vi "select edge test.vi"() -> ()   [LabVIEW 2018]
uses:
  Classes/Controller/Camera/Camera.lvclass
  <vilib>/vision/NI_Vision_Development_Module.lvlib
  <vilib>/vision/Image Controls.llb/IMAQ Image.ctl
  Classes/Controller/Camera/Material.ctl
  Classes/Controller/Camera/Camera settings.ctl
  Classes/Controller/Camera/Image processing.ctl
  Classes/Controller/Camera/Machine Vision.ctl
panel:
  out "array":sgl[](array[numeric])
  in  "Record point":bool
  out "Image Dst Out":T1
  out "Real World Coordinates":cluster{"X":sgl, "Y":sgl} {"Y" format="%.2f"; "X" format="%.2f"}
  out "Array of Real World Coordinates":cluster{"X":sgl, "Y":sgl}[](array[cluster]) {"Y" format="%.2f"; "X" format="%.2f"}
  out "Array":dbl[][](array[numeric])
  in  "Record line":bool
  in  "Stop":bool
  out "Image":T1(plugin-control)
  out "Camera":dbl[](array[numeric])
  in  "Machine Vision":T2
  in  "Image processing":T3={"Brightness"=128.0, "Contrast"=45.0, "Gamma"=1.0471123} {"Brightness" scale=0.0..400.0; "Contrast" scale=0.0..90.0; "Gamma" scale=0.005..5.0}
  in  "Camera settings":T4={"Gamma"=1.6, "Gain"=0, "Sharpness"=0, "Contrast"=0.0, "Exposure"=0.0078125} {"Exposure" min=0.000244140625 max=0.5 scale=0.0002..0.5; "Contrast" min=0.0 max=1.0 scale=0.0..1.0; "Sharpness" min=0 max=2 step=1 scale=0.0..2.0; "Gain" min=0 max=100 step=1 scale=0.0..100.0; "Gamma" min=0.01 max=10.0 scale=0.01..10.0}
  in  "Override presets":bool
  in  "Material":T5
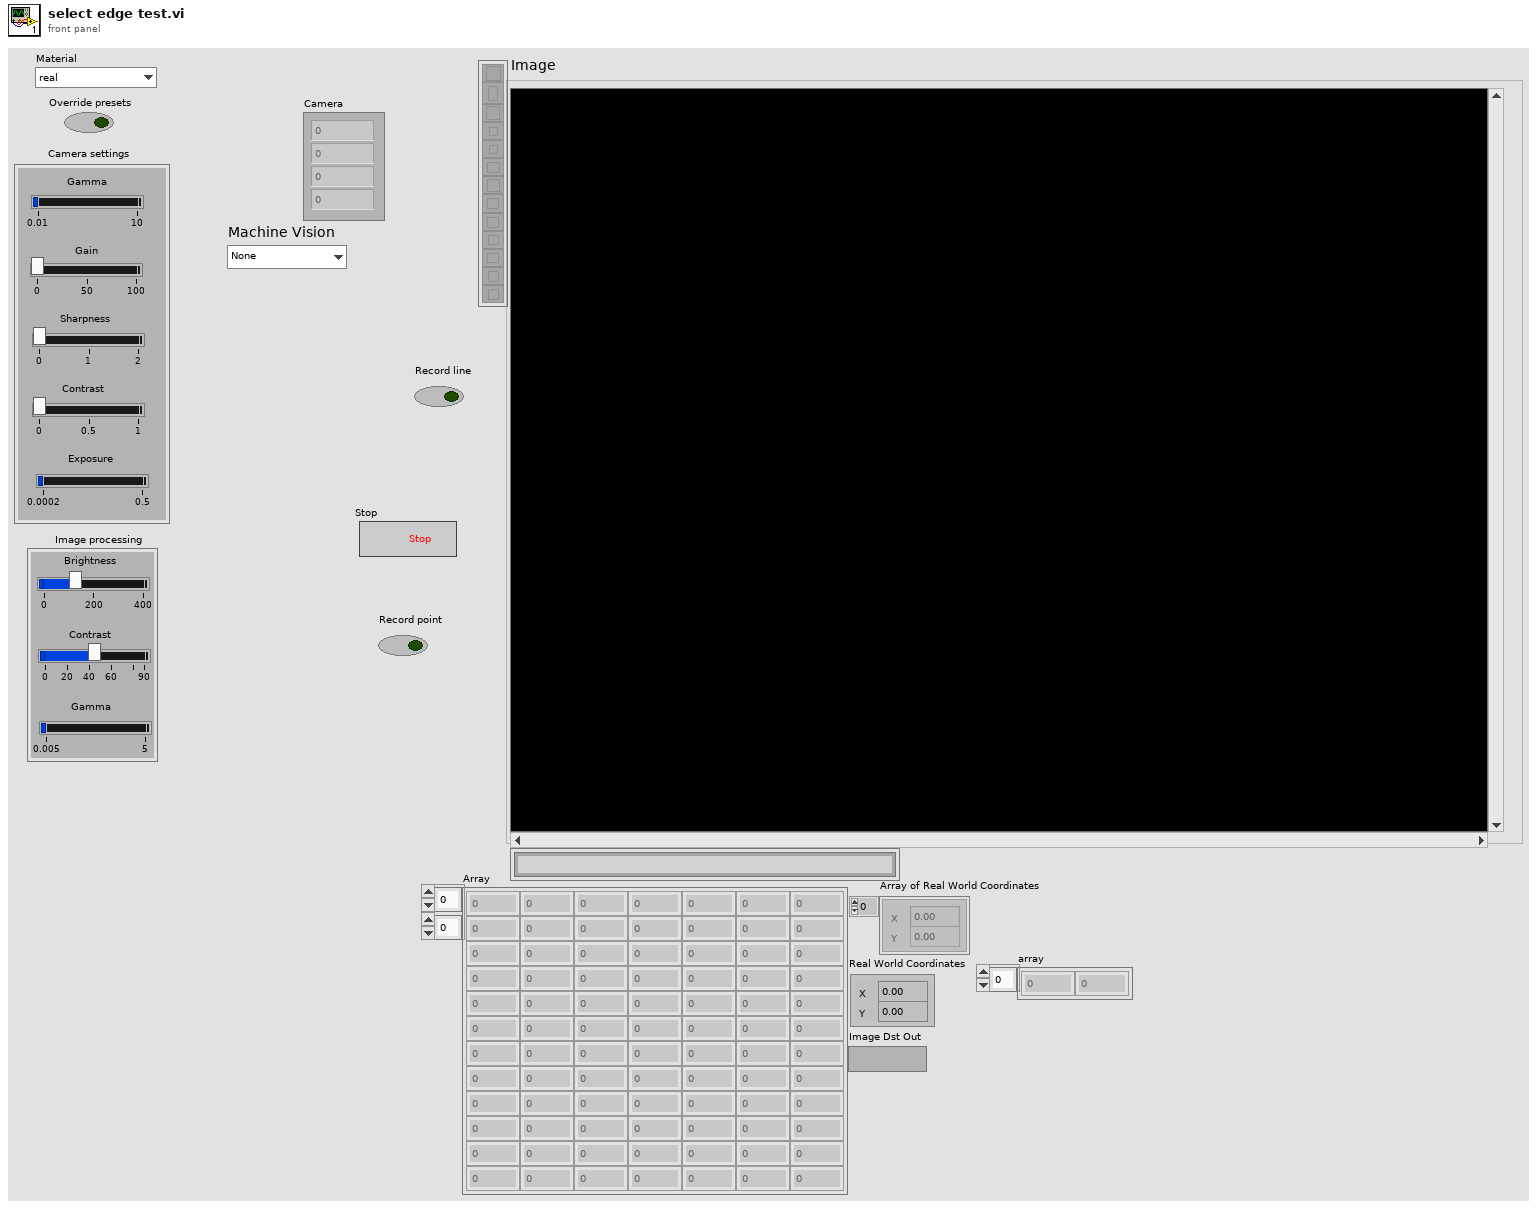
[diagram p1: front panel]
types:
  T1 = typedef "IMAQ Image.ctl" = refnum<image>
  T2 = typedef "Camera.lvclass/Machine Vision.ctl" = enum16{"None", "Tray Fiducials", "HPK Silicon", "100um dot", "Hexaboard", "Corner (TL, BR)", "Corner (BL, TR)", "BP gold pad 1", "BP gold pad 2", "BP gold pad 3", "dummy sensor CH2", "dummy sensor CH7", "dummy sensor CH191", "dummy sensor CH197", "sensor box", "sensor circle", "PCB PETG CH2", "PCB PETG CH7", "PCB PETG CH191", "PCB PETG CH197"}
  T3 = typedef "Camera.lvclass/Image processing.ctl" = cluster{"Brightness":sgl, "Contrast":sgl, "Gamma":sgl}
  T4 = typedef "Camera.lvclass/Camera settings.ctl" = cluster{"Gamma":dbl, "Gain":i64, "Sharpness":i64, "Contrast":dbl, "Exposure":dbl}
  T5 = typedef "Camera.lvclass/Material.ctl" = enum16{"real", "dummy", "PETG"}
  T6 = typedef "IMAQ Line" = cluster{"Start X":i32, "Start Y":i32, "End X":i32, "End Y":i32}
  T7 = typedef "IMAQ Point" = cluster{"X":sgl, "Y":sgl}
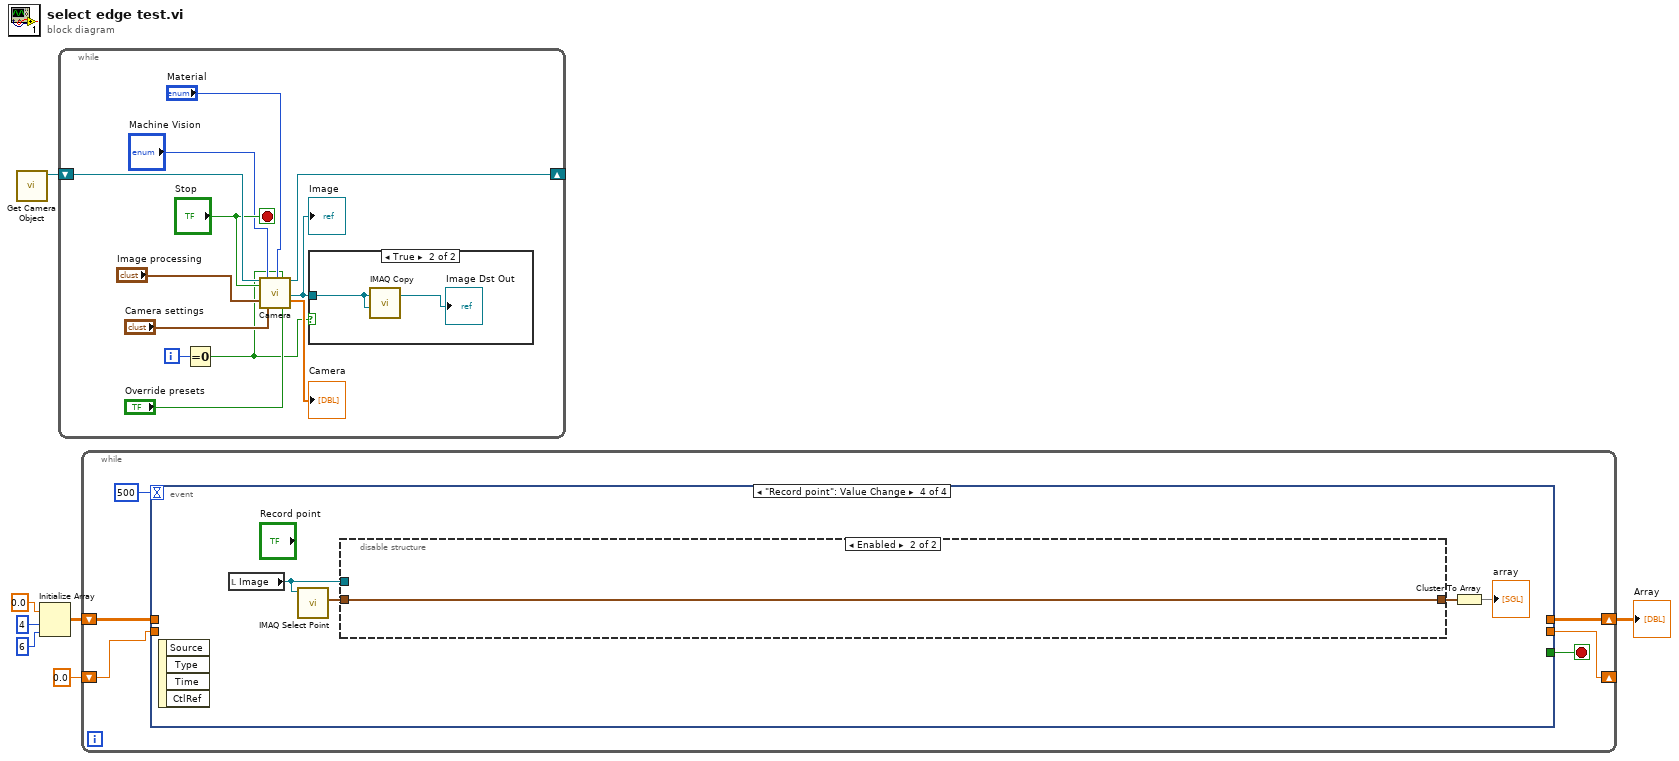
[diagram p0: block diagram]
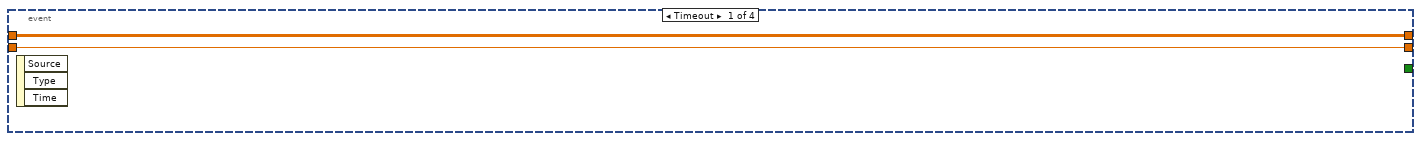
[diagram p2: hidden frame]
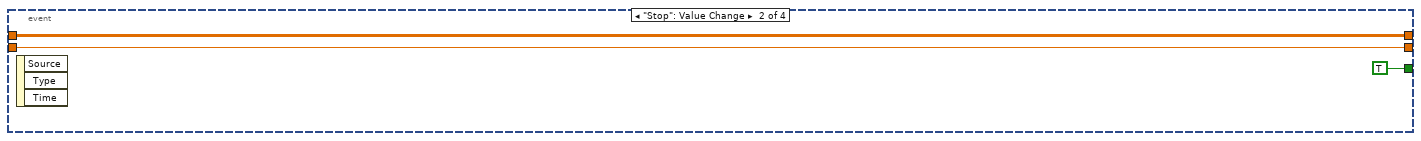
[diagram p3: hidden frame]
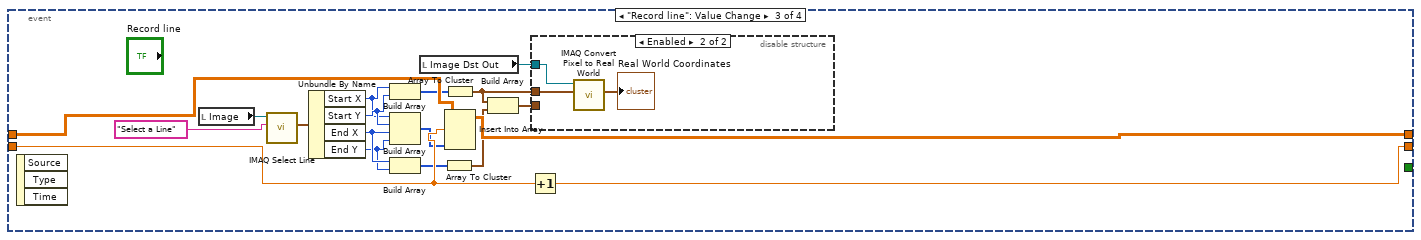
[diagram p4: hidden frame]
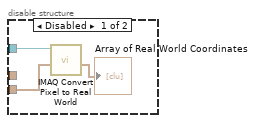
[diagram p5: hidden frame]
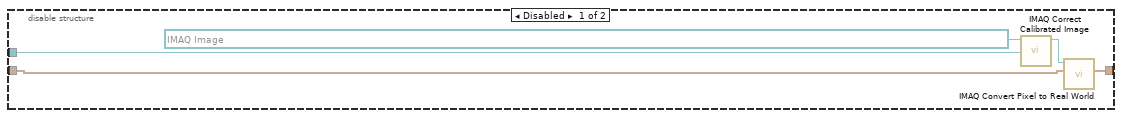
[diagram p6: hidden frame]
diagram:
  n1 = call "Get Camera Object.vi"() -> ("Camera out"=w7:refnum<class "Camera.lvclass">)  [unwired: 10 in, 1 out]
  n2 = Initialize Array(0.0 ("element"), 4 ("dimension size"), 6 ("dimension size")) -> (w6:dbl[][])
  n3 = while {
    shift-right: [w18] -> _
    shift-left: w7 -> [w19]
    i -> [w11]
    stop <- "Stop" stop-if-true
    n4 = Equal To 0?(x=w11) -> (x = 0?=w8:bool)
    n5 = call "Camera.vi"("Camera in"=w19, "Stop"="Stop", "BCG Image Processing"="Image processing", "Machine Vision"="Machine Vision", "Camera settings"="Camera settings", "Material"="Material", "Loop 0"=w8, "Override presets"="Override presets") -> ("Camera out"=w18:refnum<class "Camera.lvclass">, "Image"=w9:T1, "Camera"=→"Camera":dbl[])  [unwired: 6 in, 3 out]
    "Image" <- w9
    n6 = case shown="True" w8 {
      tunnel: w9 -> [_ w21]
      frame False {
      }
      frame True {
        n7 = call "IMAQ Copy"("Image Dst"=w21, "Image Src"=w21) -> ("Image Dst Out"=→"Image Dst Out":T1)  [unwired: 4 in, 1 out]
      }
    }
  }
  n8 = while {
    shift-right: [w25] -> _
    shift-left: 0.0 -> [w24]
    shift-right: [w23] -> w1
    shift-left: w6 -> [w26]
    stop <- w27 stop-if-true
    n9 = event shown="[3] \"Record point\": Value Change" {
      selector: _ -> [_ _ _ _]
      dyn-events: _ -> [_ _ _ _]
      timeout: 500 -> [_ _ _ _]
      tunnel: [_ TRUE _ _] -> w27
      tunnel: w26 -> [w29 w31 w50 _]
      tunnel: [w28 w30 w44 _] -> w25
      tunnel: w24 -> [w28 w30 w49 _]
      tunnel: [w29 w31 w48 _] -> w23
      event Timeout {
        n10 = event-data() -> ()  [unwired: 1 in, 3 out]
      }
      event "Stop": Value Change {
        n11 = event-data() -> ()  [unwired: 1 in, 3 out]
      }
      event "Record line": Value Change {
        n12 = event-data() -> ()  [unwired: 1 in, 3 out]
        n13 = local read "Image"() -> (w34:T1)
        n14 = call "IMAQ Select Line"("Prompt"="Select a Line", "Image In"=w34) -> ("Line"=w46:T6)  [unwired: 6 in, 3 out]
        n15 = Unbundle By Name(w46) -> ("Start X"=w42:i32, "Start Y"=w43:i32, "End X"=w39:i32, "End Y"=w38:i32)
        n16 = Build Array(w42, w43) -> (w41:i32[])
        n17 = Build Array(w42, w43, w39, w38) -> (w45:i32[])
        n18 = Build Array(w39, w38) -> (w40:i32[])
        n19 = local read "Image Dst Out"() -> (w33:T1)
        n20 = Array To Cluster(array=w40) -> (cluster=w37:cluster{"[0]":i32, "[1]":i32})
        n21 = Array To Cluster(array=w41) -> (cluster=w35:cluster{"[0]":i32, "[1]":i32})
        n22 = Insert Into Array(array=w50, index (row)=w49, new element=w45) -> (w48:dbl[][])  [unwired: 1 in]
        n23 = Build Array(w35, w37) -> (w36:cluster{"[0]":i32, "[1]":i32}[])
        n24 = Increment(x=w49) -> (x+1=w44:dbl)
        n25 = disable-structure shown="Enabled" {
          disable-tunnel: w36 -> [w53 _]
          disable-tunnel: w33 -> [w51 w54]
          disable-tunnel: w35 -> [_ w56]
          frame Disabled {
            n26 = call "IMAQ Convert Pixel to Real World"("Array of Pixel Coordinates"=w53, "Calibrated Image"=w51) -> ("Array of Real World Coordinates"=→"Array of Real World Coordinates":cluster{"X":sgl, "Y":sgl}[])  [unwired: 4 in, 5 out]
          }
          frame Enabled {
            n27 = call "IMAQ Convert Pixel to Real World"("Pixel Coordinates"=w56, "Calibrated Image"=w54) -> ("Real World Coordinates"=→"Real World Coordinates":cluster{"X":sgl, "Y":sgl})  [unwired: 4 in, 5 out]
          }
        }
      }
      event "Record point": Value Change {
        n28 = event-data() -> ()  [unwired: 1 in, 4 out]
        n29 = local read "Image"() -> (w57:T1)
        n30 = call "IMAQ Select Point"("Image In"=w57) -> ("Point"=w60:T7)  [unwired: 7 in, 3 out]
        n31 = disable-structure shown="Enabled" {
          disable-tunnel: w60 -> [w65 w66]
          disable-tunnel: [w64 w66] -> w59
          disable-tunnel: w57 -> [w63 _]
          frame Disabled {
            n32 = call "IMAQ Correct Calibrated Image"("Image Dst"=w63, "Image Src"=T1 refnum) -> ("Corrected Image"=w61:T1)  [unwired: 8 in, 1 out]
            n33 = call "IMAQ Convert Pixel to Real World"("Pixel Coordinates"=w65, "Calibrated Image"=w61) -> ("Real World Coordinates"=w64:cluster{"X":sgl, "Y":sgl})  [unwired: 4 in, 5 out]
          }
          frame Enabled {
          }
        }
        n34 = Cluster To Array(cluster=w59) -> (array=→"array":sgl[])
      }
    }
  }
  "Array" <- w1
